vi "Read PAE Pins.vi"(8 "error in (no error)":errorcluster, 11 "QPA Measurement in":refnum<class "QPA Measurement.lvclass">=refnum) -> (0 "error out":errorcluster, 2 "PAE Pins":string[](array[string]), 3 "QPA Measurement out":refnum<class "QPA Measurement.lvclass">)   [LabVIEW 2016, in "QPA Measurement.lvlib" / "QPA Measurement.lvclass"]
uses:
  QPA Measurement.lvclass
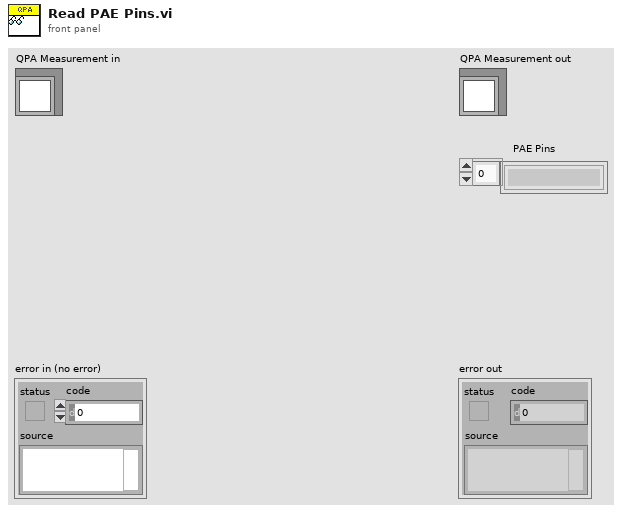
[diagram p1: front panel]
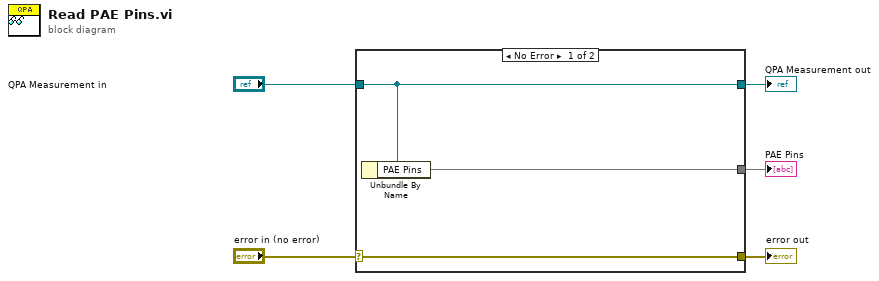
[diagram p0: block diagram]
diagram:
  n1 = case shown="No Error" "error in (no error)" {
    selector: "error in (no error)" -> [w8 w9]
    tunnel: [w8 w9] -> w4
    tunnel: [w7 w10] -> w2
    tunnel: "QPA Measurement in" -> [w7 w10]
    tunnel: [w6 _] -> w1
    frame No Error {
      n2 = Unbundle By Name(w7) -> ("PAE Pins"=w6)
    }
    frame Error {
    }
  }
  "error out" <- w4
  "QPA Measurement out" <- w2
  "PAE Pins" <- w1
